vi "Get Cell Data[i].vi"(8 "error in (no error)":errorcluster, 11 "PAS in":refnum<class "PAS.lvclass">) -> (0 "error out":errorcluster, 2 "Cell Data[i]":refnum<class "PAS Cell Data.lvclass">, 3 "PAS out":refnum<class "PAS.lvclass">)   [LabVIEW 2014, in "PAS.lvclass"]
uses:
  PAS.lvclass
  Data/Cell/PAS Cell Data.lvclass
  PAS.lvclass/PAS.ctl
  Data/Main/PAS Data.lvclass
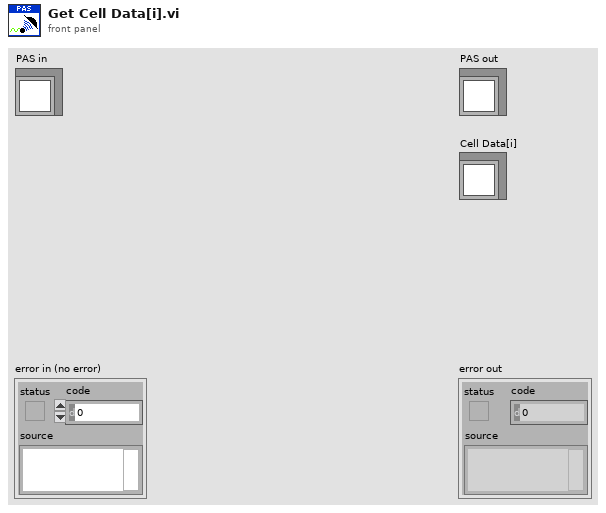
[diagram p1: front panel]
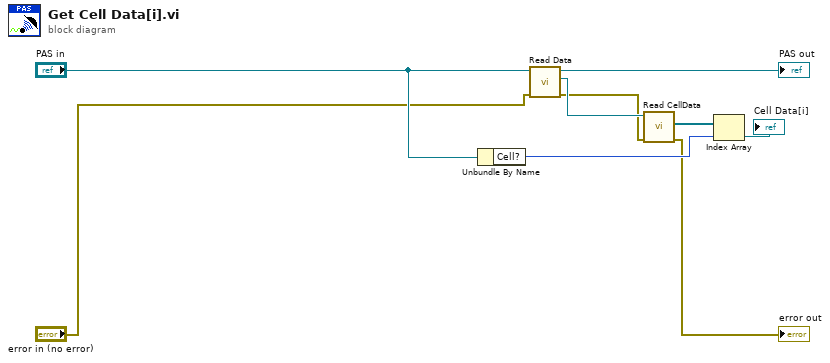
[diagram p0: block diagram]
diagram:
  n1 = Unbundle By Name("PAS in") -> ("Cell?"=w6:i32)
  n2 = call "Read Data.vi"("error in"="error in (no error)", "PAS in"="PAS in") -> ("error out"=w2:errorcluster, "PAS Data.lvclass"=w7:refnum<class "PAS Data.lvclass">, "PAS out"=→"PAS out":refnum<class "PAS.lvclass">)  [unwired: 7 in]
  n3 = call "Read CellData.vi"("error in"=w2, "PAS Data in"=w7) -> ("error out"=→"error out":errorcluster, "CellData"=w5:refnum<class "PAS Cell Data.lvclass">[])  [unwired: 7 in, 1 out]
  n4 = Index Array(array=w5, index=w6) -> (element=→"Cell Data[i]":refnum<class "PAS Cell Data.lvclass">)
